vi "AIP Write Depth Min.vi"(8 "error in (no error)":errorcluster, 10 "Depth":dbl, 11 "AIP Instrument in":refnum<class "AIP Instrument.lvclass">) -> (0 "error out":errorcluster, 3 "AIP Instrument out":refnum<class "AIP Instrument.lvclass">)   [LabVIEW 2015, in "AIP Instrument.lvlib" / "AIP Instrument.lvclass"]
uses:
  AIP Instrument.lvclass
  AIP Instrument.lvclass/AIP Instrument.ctl
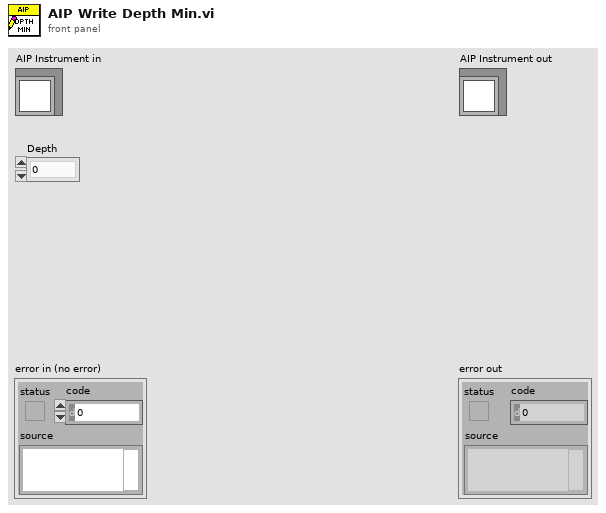
[diagram p1: front panel]
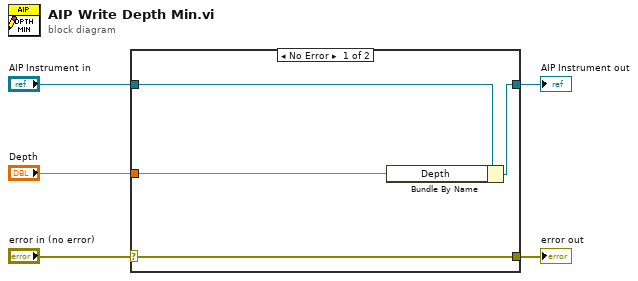
[diagram p0: block diagram]
diagram:
  n1 = case shown="No Error" "error in (no error)" {
    selector: "error in (no error)" -> [w9 w10]
    tunnel: [w9 w10] -> w4
    tunnel: [w7 w11] -> w2
    tunnel: "AIP Instrument in" -> [w8 w11]
    tunnel: "Depth" -> [w6 _]
    frame No Error {
      n2 = Bundle By Name(cluster=w8, "Depth"=w6) -> (w7:refnum<class "AIP Instrument.lvclass">)
    }
    frame Error {
    }
  }
  "error out" <- w4
  "AIP Instrument out" <- w2
